vi "GetLibTemplates.vi"(0 "LibWriter":refnum<class "LibWriter.lvclass">, 1 "DerivedFromThisLib(if any)":refnum<vi>, 5 "error in (no error)":errorcluster) -> (14 "LibWriter":refnum<class "LibWriter.lvclass">, 15 "Templates":T1[](array[typedef]), 19 "error out":errorcluster)   [LabVIEW 2014, in "LibWriter.lvclass"]
uses:
  <resource>/Framework/Providers/Open_GDS/ClassProviders/LibProvider_BaseClassInterface/LibWriter_class/ClassWriter_class/LibWriter.lvclass
  <resource>/Framework/Providers/Open_GDS/ClassProviders/LibProvider_BaseClassInterface/LibWriter_class/LibTemplateType.vi
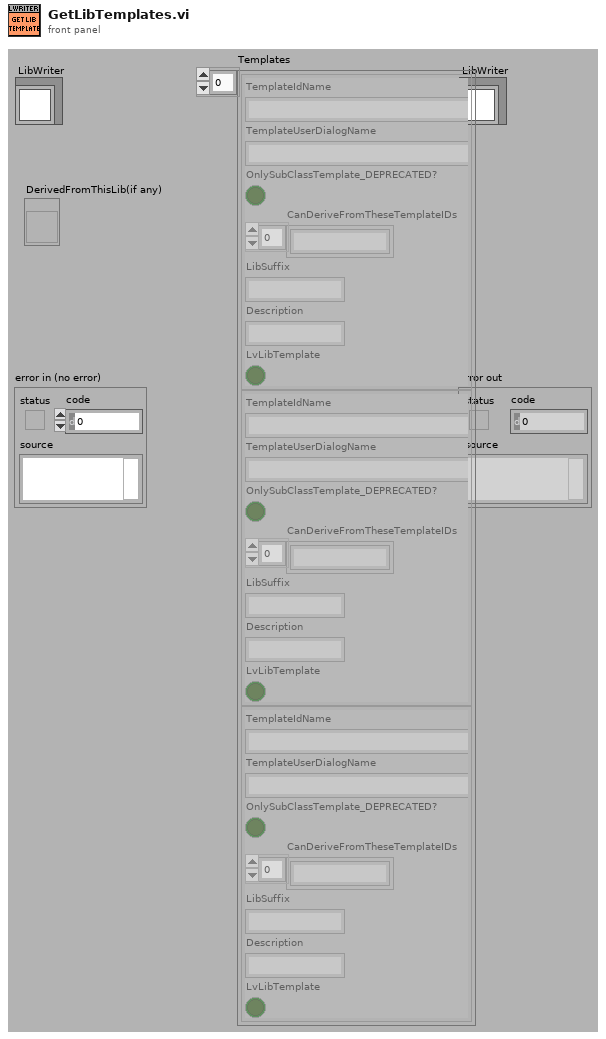
[diagram p1: front panel]
types:
  T1 = typedef "LibWriter.lvclass/LibTemplateType.vi" = cluster{"TemplateIdName":string, "TemplateUserDialogName":string, "OnlySubClassTemplate_DEPRECATED?":bool, "CanDeriveFromTheseTemplateIDs":string[], "LibSuffix":string, "Description":string, "LvLibTemplate":bool}
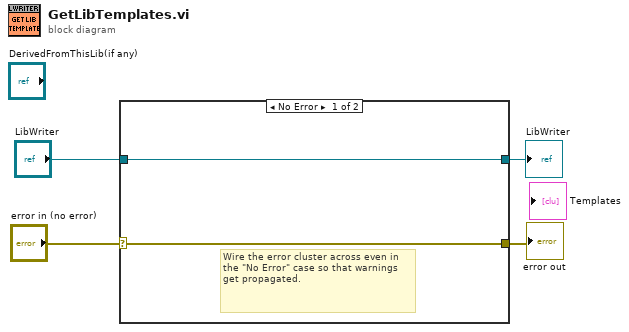
[diagram p0: block diagram]
diagram:
  n1 = case shown="No Error" "error in (no error)" {
    selector: "error in (no error)" -> [w5 w8]
    tunnel: [w5 w8] -> w3
    tunnel: [w6 w7] -> w1
    tunnel: "LibWriter" -> [w6 w7]
    frame No Error {
      # "Wire the error cluster across even in the \"No Error\" case so that warnings get propagated."
    }
    frame Error {
    }
  }
  "error out" <- w3
  "LibWriter" <- w1
